vi "Read Font.vi"(8 "error in (no error)":errorcluster, 11 "PDF Report Class in":refnum<class "PDF Report Class.lvclass">) -> (0 "error out":errorcluster, 2 "Font Class.lvclass":refnum<class "Font Class.lvclass">, 3 "PDF Report Class out":refnum<class "PDF Report Class.lvclass">)   [LabVIEW 2019, in "PDF Report Class.lvclass"]
uses:
  <userlib>/Exaprom PDF/LV Class/PDF Report Class/PDF Report Class.lvclass
  <userlib>/Exaprom PDF/LV Class/Fonts Class/Font Class.lvclass
  <userlib>/Exaprom PDF/LV Class/PDF Report Class/PDF Report Class.lvclass/PDF Report Class.ctl
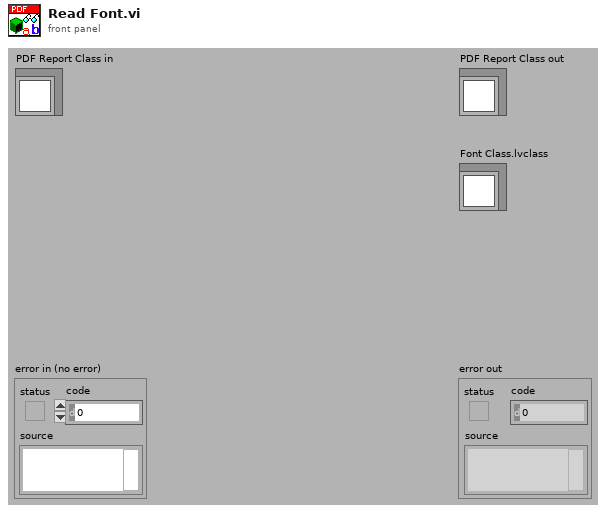
[diagram p1: front panel]
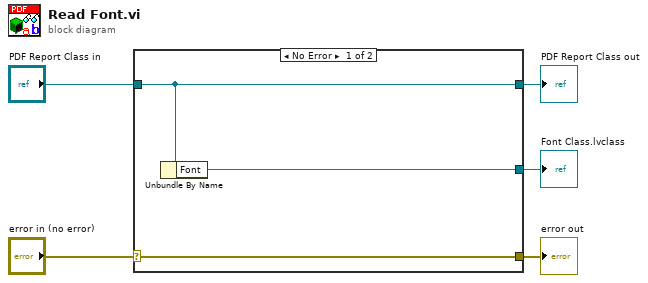
[diagram p0: block diagram]
diagram:
  n1 = case shown="No Error" "error in (no error)" {
    selector: "error in (no error)" -> [w8 w9]
    tunnel: [w8 w9] -> w4
    tunnel: [w7 w10] -> w2
    tunnel: "PDF Report Class in" -> [w7 w10]
    tunnel: [w6 _] -> w1
    frame No Error {
      n2 = Unbundle By Name(w7) -> ("Font"=w6:refnum<class "Font Class.lvclass">)
    }
    frame Error {
    }
  }
  "error out" <- w4
  "PDF Report Class out" <- w2
  "Font Class.lvclass" <- w1
